vi "Temp_Schedule.vi"(10 "First Time?":bool) -> (3 "?":cluster{"time (s)":dbl, "setpoint":dbl}[](array[cluster]))   [LabVIEW 2009]
panel:
  in  "?":cluster{"time (s)":dbl, "setpoint":dbl}[](array[cluster])
  in  "Done":bool
  # "Choose a Temperature Schedule:\nIt is up to the user to make sure that time and temperature values are valid.  This includes:\n  -  The first time value is 0 s.\n  -  Time values are in order from smallest to largest.\n  -  Temperatures are within system limits (e.g. greater than room temperature).\n  -  Ramp rates are not too high."
  # "Time [s]"
  # "Temperature [C]"
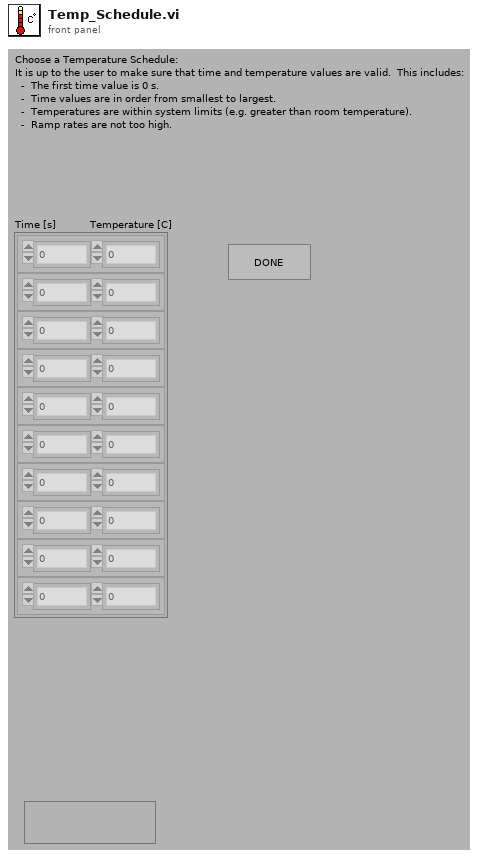
[diagram p1: front panel]
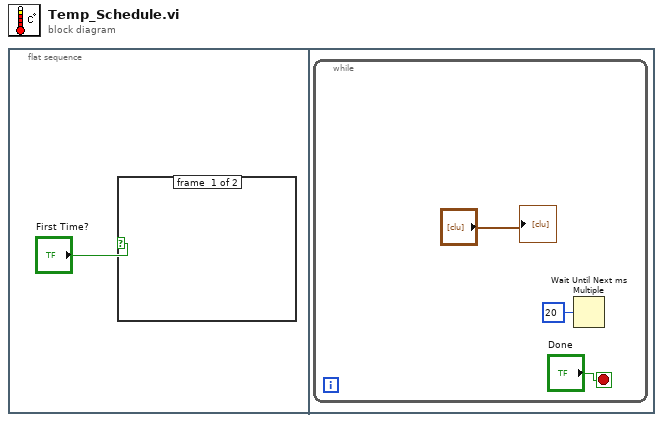
[diagram p0: block diagram]
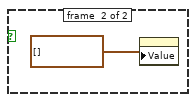
[diagram p2: hidden frame]
diagram:
  n1 = flat-sequence {
    frame #0 {
      n2 = case shown="True" "First Time?" {
        frame #0 {
        }
        frame #1 {
          n3 = property class="Arr (strict)"("Value"=cluster{"time (s)":dbl, "setpoint":dbl}[] []) -> ()  [unwired: 2 in, 2 out]
        }
      }
    }
    frame #1 {
      n4 = while {
        stop <- "Done" stop-if-true
        n5 = Wait Until Next ms Multiple(millisecond multiple=u32 20) -> ()  [unwired: 1 out]
        "?" <- "?"
      }
    }
  }
